vi "Themes.vi"(11 "Theme Choice":T1) -> (1 "Text":u32, 2 "Accent":u32, 3 "BG Color":u32, 4 "Accent2":u32)   [LabVIEW 2019, in "LSS.lvlib"]
doc: "This VI outputs the style settings specified by the Theme Choice.\n\n<b>Inputs:</b>\n<b>Theme Choice</b> - Select theme that will be output.\n\n<b>Outputs:</b>\n<b>BG Color</b> - Background color of the selected theme.\n<b>Accent</b> - Accent color of the selected theme\n<b>Text</b> - Font color for selected theme\n<b>Accent2</b> - Second accent color for selected theme."
uses:
  LSS.lvlib
  Themes.ctl
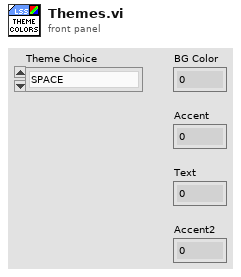
[diagram p1: front panel]
types:
  T1 = typedef "LSS.lvlib/Themes.ctl" = enum16{"SPACE", "ATK", "THEME1", "THEME2"}
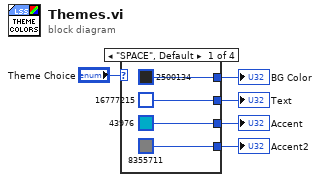
[diagram p0: block diagram]
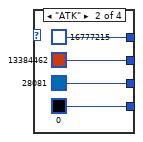
[diagram p2: hidden frame]
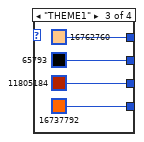
[diagram p3: hidden frame]
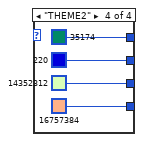
[diagram p4: hidden frame]
diagram:
  n1 = case shown="\"SPACE\", Default" "Theme Choice" {
    tunnel: [u32 43976 u32 28081 u32 11805184 u32 14352312] -> w2
    tunnel: [u32 2500134 u32 16777215 u32 16762760 u32 35174] -> w3
    tunnel: [u32 16777215 u32 13384462 u32 65793 u32 220] -> w4
    tunnel: [u32 8355711 u32 0 u32 16737792 u32 16757384] -> w5
    frame "SPACE", Default {
    }
    frame "ATK" {
    }
    frame "THEME1" {
    }
    frame "THEME2" {
    }
  }
  "Accent2" <- w5
  "Text" <- w4
  "BG Color" <- w3
  "Accent" <- w2
